vi "Create Class.vi"(8 "error in (no error)":errorcluster, 11 "Message Maker in":refnum<class "Concrete Message Rescripter.lvclass">) -> (0 "error out":errorcluster, 3 "Message Maker out":refnum<class "Concrete Message Rescripter.lvclass">)   [LabVIEW 2020, in "Message Rescripter.lvlib" / "Concrete Message Rescripter.lvclass"]
uses:
  Concrete Message Rescripter.lvclass
  <vilib>/Utility/EditLVLibs/Edit LVLibs.lvlib
  MessageMakerProvider/_Message Maker/_Maker Classes/Message Scripter/Message Scripter.lvclass
  Message Rescripter.lvlib
  <vilib>/Utility/traverseref.llb/TRef TravTarget.ctl
  MessageMakerProvider/_Message Maker/Message Maker.lvlib
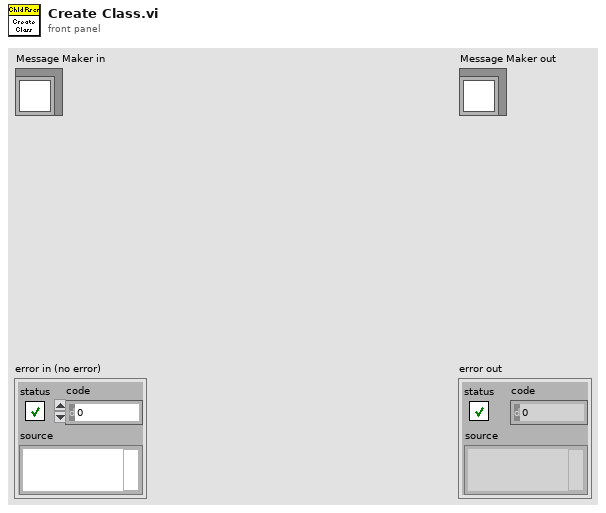
[diagram p1: front panel]
types:
  T1 = typedef "TRef TravTarget.ctl" = enum16{"FP", "BD", "Other"}
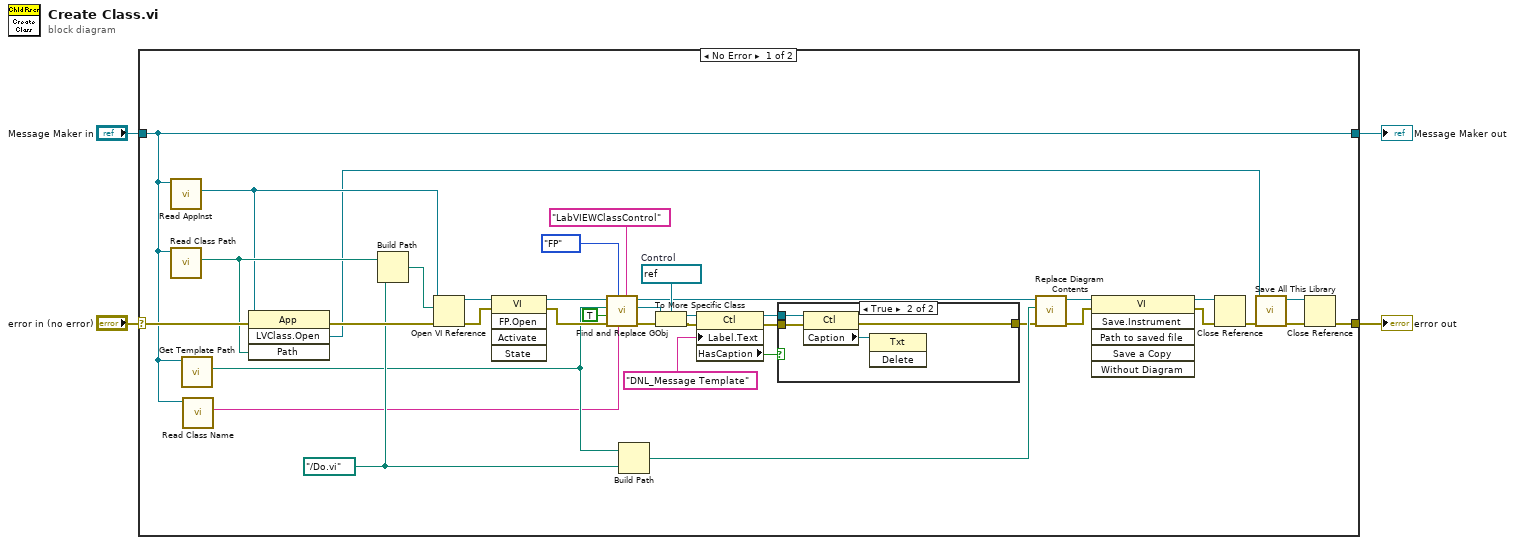
[diagram p0: block diagram]
diagram:
  n1 = case shown="No Error" "error in (no error)" {
    selector: "error in (no error)" -> [w37 w48]
    tunnel: [w38 w48] -> w1
    tunnel: [w16 w47] -> w2
    tunnel: "Message Maker in" -> [w16 w47]
    frame No Error {
      w20 = path "../Do.vi"
      w21 = refnum<vi> refnum  # Control
      n2 = call "Read AppInst.vi"("Message Maker in"=w16) -> ("AppInst"=w18:refnum<vi>)  [unwired: 10 in]
      n3 = call "Read Class Path.vi"("Message Scripter in"=w16) -> ("Class Path"=w35:path)  [unwired: 10 in]
      n4 = call-dynamic "Get Template Path.vi"("Concrete Message Scripter in"=w16) -> ("Template Path"=w19:path)  [unwired: 10 in]
      n5 = call "Read Class Name.vi"("Message Scripter in"=w16) -> ("Class Name"=w15:string)  [unwired: 10 in]
      n6 = invoke class="App" method="LVClass.Open"(reference=w18, error in=w37, "Path"=w35) -> (error out=w41:errorcluster, "LVClass.Open"=w17:refnum<vi>)  [unwired: 1 in, 2 out]
      n7 = Build Path(base path=w35, name or relative path=w20) -> (appended path=w34:path)
      n8 = Open VI Reference(application reference (local)=w18, vi path=w34, error in (no error)=w41) -> (vi reference=w30:refnum<vi>, error out=w28:errorcluster)  [unwired: 3 in]
      n9 = invoke class="VI" method="FP.Open"(reference=w30, error in=w28) -> (reference out=w29:refnum<vi>, error out=w27:errorcluster)  [unwired: 3 in, 3 out]
      n10 = call "Find and Replace GObj.vi"("GObj Class Name"="LabVIEWClassControl", "GObj Label"=w15, "Traverse Target"=TRef_TravTarget."FP", "error in (no error)"=w27, "Case Insensitive Match? (F)"=TRUE, "Class Path"=w19, "vi reference in"=w29) -> ("error out"=w22:errorcluster, "Replace"=w8:refnum<vi>, "vi reference out"=w6:refnum<vi>)  [unwired: 2 in]
      n11 = Build Path(base path=w19, name or relative path=w20) -> (appended path=w31:path)
      n12 = To More Specific Class(target class=w21, reference=w8, error in=w22) -> (specific class reference=w7:refnum<vi>, error out=w9:errorcluster)
      n13 = property class="Ctl"(reference=w7, error in=w9, "Label.Text"="DNL_Message Template") -> (reference out=w11:refnum<vi>, error out=w12:errorcluster, "HasCaption"=w13:bool)
      n14 = case shown="True" w13 {
        tunnel: w11 -> [_ w45]
        tunnel: w12 -> [w42 w44]
        tunnel: [w42 w43] -> w10
        frame False {
        }
        frame True {
          n15 = property class="Ctl"(reference=w45, error in=w44) -> (error out=w43:errorcluster, "Caption"=w46:refnum<vi>)  [unwired: 1 out]
          n16 = invoke class="Txt" method="Delete"(reference=w46) -> ()  [unwired: 2 in, 3 out]
        }
      }
      n17 = call "Replace Diagram Contents.vi"("error in (no error)"=w10, "Template VI"=w31, "Target VI"=w6) -> ("error out"=w32:errorcluster, "dup Target VI"=w33:refnum<vi>)  [unwired: 7 in]
      n18 = invoke class="VI" method="Save.Instrument"(reference=w33, error in=w32) -> (reference out=w26:refnum<vi>, error out=w25:errorcluster)  [unwired: 4 in, 4 out]
      n19 = Close Reference(reference=w26, error in (no error)=w25) -> (error out=w40:errorcluster)
      n20 = call <vilib>:"Save All This Library.vi"("error in (no error)"=w40, "Library in"=w17) -> ("error out"=w39:errorcluster, "Library out"=w36:refnum<vi>)  [unwired: 8 in]
      n21 = Close Reference(reference=w36, error in (no error)=w39) -> (error out=w38:errorcluster)
    }
    frame Error {
    }
  }
  "error out" <- w1
  "Message Maker out" <- w2
